vi "Voltage - Continuous Input.vi"() -> ()   [LabVIEW 2014]
doc: "이 예는 DAQmx 디바이스를 사용하여 버퍼링된 전압 측정을 연속적으로 수집하는 방법을 보여줍니다.\n\nDAQ 디바이스에 신호를 연결하는 방법에 대한 설명은 해당 디바이스 문서를 참조하십시오."
uses:
  <vilib>/DAQmx/create/channels.llb/DAQmx Create Channel (AI-Voltage-Basic).vi
  <vilib>/DAQmx/configure/timing.llb/DAQmx Timing (Sample Clock).vi
  <vilib>/DAQmx/configure/task.llb/DAQmx Configure Logging (TDMS).vi
  <vilib>/DAQmx/read.llb/DAQmx Read (Analog 1D Wfm NChan NSamp).vi
  <resource>/objmgr/daqmx.rc
panel:
  in  "정지":bool
  out "웨이브폼 그래프":waveform(dbl)[](graph)
  in  "TDMS파일 경로":path
  in  "루프당 샘플":i32=1000
  in  "샘플 속도":dbl=1000.0
  in  "샘플 클럭 소스":tag="OnboardClock"
  in  "터미널 설정":i32(ring)=-1 items=["기본"=-1, "RSE"=10083, "NRSE"=10078, "차동"=10106, "유사 차동"=12529]
  in  "최대 전압":dbl=5.0
  in  "최소 전압":dbl=-5.0
  in  "물리적 채널":tag="Dev1/ai0"
  out "실제 샘플 속도":dbl=1000.0 format="%0.2f"
  in  "로깅 모드":i32(ring)=10231 items=["Off"=10231, "로그 및 읽기"=15842]
  # "채널 셋팅"
  # "수집된 데이터"
  # "타이밍 셋팅"
  # "로깅 셋팅"
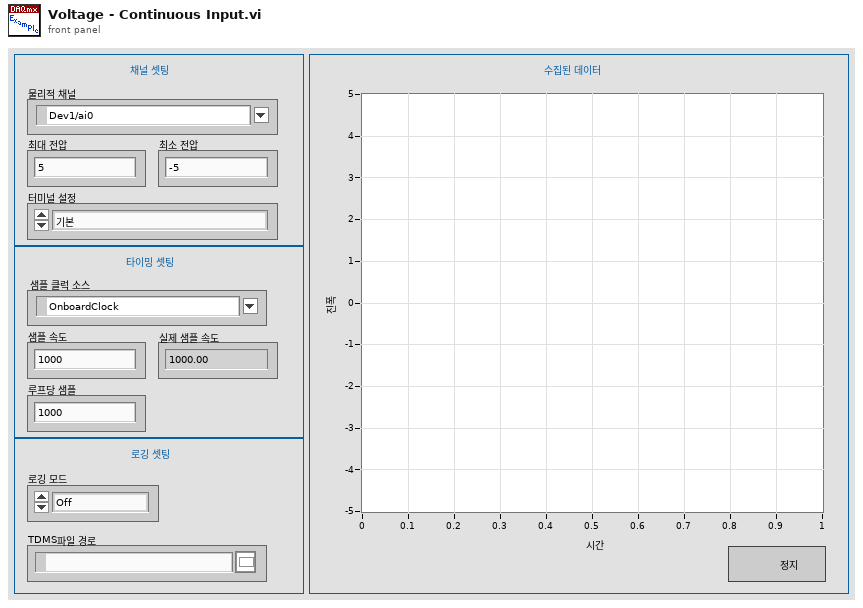
[diagram p1: front panel]
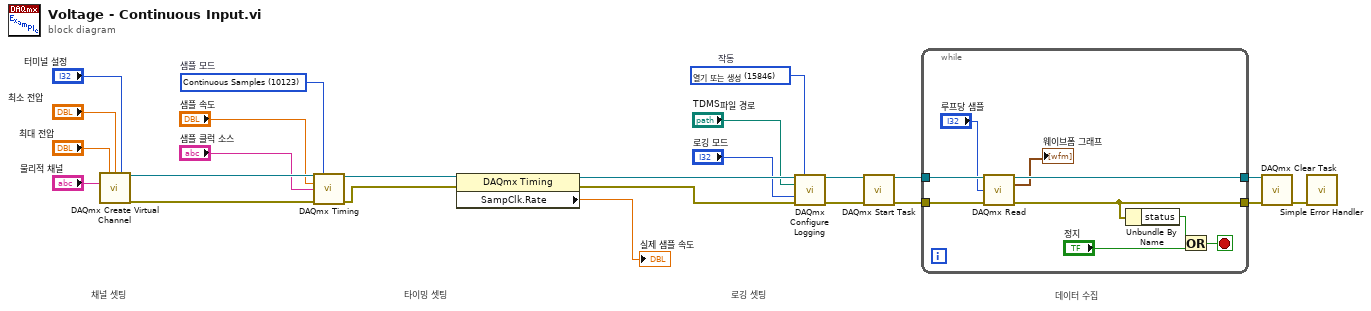
[diagram p0: block diagram]
diagram:
  w17 = 15846 items=["Open"=10437, "열기 또는 생성"=15846, "생성 또는 대체"=15847, "생성"=15848]  # 작동
  w22 = 10123 items=["유한 샘플"=10178, "Continuous Samples"=10123, "하드웨어 타이밍에 의한 단일 포인트"=12522]  # 샘플 모드
  # "데이터 수집"
  # "타이밍 셋팅"
  # "채널 셋팅"
  # "로깅 셋팅"
  n1 = call-poly <vilib>:"DAQmx Create Virtual Channel.vi"("maximum value"="최대 전압", "minimum value"="최소 전압", "input terminal configuration"="터미널 설정", "physical channels"="물리적 채널") -> ("task out"=w20:refnum<k21>, "error out"=w21:errorcluster)  [unwired: 10 in]
  n2 = call-poly <vilib>:"DAQmx Timing.vi"("task/channels in"=w20, "sample mode"=w22, "rate"="샘플 속도", "source"="샘플 클럭 소스", "error in"=w21) -> ("task out"=w24:refnum<k21>, "error out"=w23:errorcluster)  [unwired: 9 in]
  n3 = property class="DAQmx Timing"(reference=w24, error in=w23) -> (reference out=w19:refnum<k21>, error out=w18:errorcluster, "SampClk.Rate"=→"실제 샘플 속도":dbl)
  n4 = call-poly <vilib>:"DAQmx Configure Logging.vi"("task/channels in"=w19, "operation"=w17, "file path"="TDMS파일 경로", "logging mode"="로깅 모드", "error in"=w18) -> ("task out"=w2:refnum<k21>, "error out"=w1:errorcluster)  [unwired: 9 in]
  n5 = call <vilib>:"DAQmx Start Task.vi"("task/channels in"=w2, "error in"=w1) -> ("task out"=w16:refnum<k21>, "error out"=w15:errorcluster)  [unwired: 12 in]
  n6 = while {
    tunnel: w16 -> [w33]
    tunnel: w15 -> [w32]
    tunnel: [w29] -> w13
    tunnel: [w30] -> w14
    stop <- w31 stop-if-true
    n7 = call-poly <vilib>:"DAQmx Read.vi"("task/channels in"=w33, "number of samples per channel"="루프당 샘플", "error in"=w32) -> ("task out"=w30:refnum<k21>, "data"=→"웨이브폼 그래프":waveform(dbl)[], "error out"=w29:errorcluster)  [unwired: 10 in]
    n8 = Unbundle By Name(w29) -> ("status"=w28:bool)
    n9 = Or(x=w28, y="정지") -> (x .or. y?=w31:bool)
  }
  n10 = call <vilib>:"DAQmx Clear Task.vi"("task in"=w14, "error in"=w13) -> ("error out"=w12:errorcluster)  [unwired: 13 in]
  n11 = call <vilib>:"Simple Error Handler.vi"("error in (no error)"=w12) -> ()  [unwired: 4 in, 5 out]
